vi "hashFN.vi"(4 "DWORD":u32 format="%08x") -> (1 "hash":string="2DC0180030")   [LabVIEW 2015]
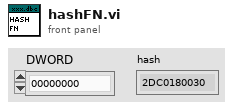
[diagram p1: front panel]
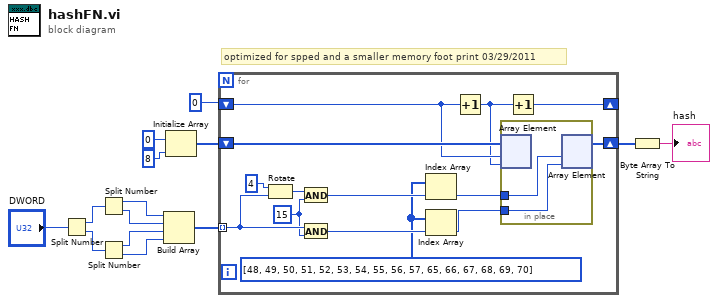
[diagram p0: block diagram]
diagram:
  # "optimized for spped and a smaller memory foot print 03/29/2011"
  n1 = Split Number(x="DWORD") -> (hi(x)=w12:u16, lo(x)=w13:u16)
  n2 = Split Number(x=w12) -> (hi(x)=w8:u8, lo(x)=w11:u8)
  n3 = Split Number(x=w13) -> (hi(x)=w10:u8, lo(x)=w9:u8)
  n4 = Build Array(w8, w11, w10, w9) -> (w2:u8[])
  n5 = Initialize Array(u8 0, 8 ("y")) -> (w5:u8[])
  n6 = for {
    tunnel: w2 -> [w28] mode=indexing
    shift-right: [w23] -> w6
    shift-left: w5 -> [w24]
    shift-right: [w16] -> _
    shift-left: 0 -> [w17]
    w20 = u8[] [48, 49, 50, 51, 52, 53, 54, 55, 56, 57, 65, 66, 67, 68, 69, 70] ("byte Array")
    w26 = u8 15 ("y")
    n7 = Rotate(1:w28, 2:i8 4 ("y")) -> (0:w25:u8)
    n8 = And(x=w25, y=w26) -> (x .and. y?=w22:u8)
    n9 = And(x=w28, y=w26) -> (x .and. y?=w21:u8)
    n10 = Index Array(array=w20, index=w22) -> (element=w19:u8)
    n11 = Index Array(array=w20, index=w21) -> (element=w18:u8)
    n12 = Increment(x=w17) -> (x+1=w15:i32)
    n13 = in-place {
      in-place-border: w19 -> [w30]
      in-place-border: w18 -> [w29]
      n14 = in-place-array #1(w24, w17, w15) -> ()  [unwired: 2 out]
      n15 = in-place-array #1(w30, w29) -> (w23:u8[])  [unwired: 2 out]
    }
    n16 = Increment(x=w15) -> (x+1=w16:i32)
  }
  n17 = Byte Array To String(unsigned byte array=w6) -> (string=→"hash":string)
